vi "Configure Output Filter External.vi"(7 "Enable External Filter (F: Disable)":bool, 8 "error in (no error)":errorcluster, 9 "External Filter Type (1: Ultra Low Noise Filter)":i32(ring)=1 items=["Low Noise Filter", "Ultra Low Noise Filter", "High Current Ultra Low Noise Filter"], 10 "Output Channel (0: Channel 1)":i32(ring) items=["Channel 1", "Channel 2"], 11 "VISA resource name":refnum<visa-resource-name>) -> (0 "error out":errorcluster, 3 "VISA resource name out":refnum<visa-resource-name>)   [LabVIEW 2026, in "Agilent B2900 Series.lvlib"]
doc: "Configure the output external filter.\n\n<B>Note:</B>\nThis VI is only supported by Agilent models B2961A, B2962A. B2961B, B2962B, B2961C and B2962C."
uses:
  Agilent B2900 Series.lvlib
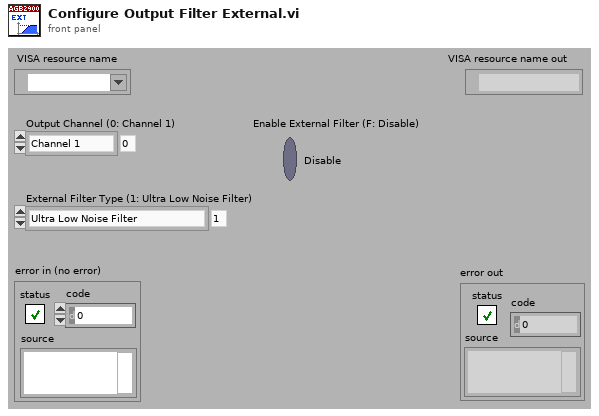
[diagram p1: front panel]
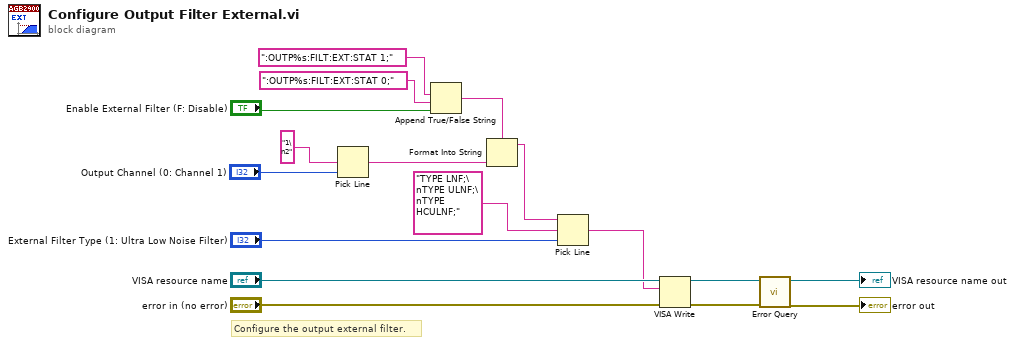
[diagram p0: block diagram]
diagram:
  # "Configure the output external filter."
  n1 = Pick Line(multi-line string="1\n2" ("string (\"\")"), line index="Output Channel (0: Channel 1)") -> (output string=w3:string)  [unwired: 1 in]
  n2 = Append True/False String(1:"Enable External Filter (F: Disable)", 2:":OUTP%s:FILT:EXT:STAT 0;", 3:":OUTP%s:FILT:EXT:STAT 1;") -> (0:w4:string)  [unwired: 1 out]
  n3 = Format Into String(format string=w4, w3) -> (resulting string=w2:string)  [unwired: 2 in, 1 out]
  n4 = Pick Line(string ("")=w2, multi-line string="TYPE LNF;\nTYPE ULNF;\nTYPE HCULNF;", line index="External Filter Type (1: Ultra Low Noise Filter)") -> (output string=w1:string)
  n5 = VISA Write(VISA resource name="VISA resource name", write buffer=w1, error in (no error)="error in (no error)") -> (VISA resource name out=w13:refnum<visa-resource-name>, error out=w12:errorcluster)  [unwired: 1 out]
  n6 = call "Error Query.vi"("error in (no error)"=w12, "VISA resource name"=w13) -> ("error out"=→"error out":errorcluster, "VISA resource name out"=→"VISA resource name out":refnum<visa-resource-name>)  [unwired: 8 out]
